vi "Get Control Offsets by Name.vi"(6 "offset":i32, 8 "error in (no error)":errorcluster, 9 "Controls":string[](array[string]), 10 "Indicators":string[](array[string]), 11 "bitfile xml in":string) -> (0 "error out":errorcluster, 1 "Control Offsets":T1[](array[typedef]), 2 "Indicator Offsets":T1[](array[typedef]), 4 "offset past EndTag":i32)   [LabVIEW 2010, in "FPGA Bitfile Utility.lvlib"]
uses:
  <userlib>/_FPGA Interface Advanced Tools/FPGA Bitfile Utility/FPGA Bitfile Utility.lvlib
  <userlib>/_FPGA Interface Advanced Tools/FPGA Bitfile Utility/TypeDefs/Control_Indicator Info.ctl
  <vilib>/rvi/DataTransferAndStorage/Container/Common/niFpgaDataTypeControl.ctl
  <userlib>/_FPGA Interface Advanced Tools/FPGA Bitfile Utility/Get Register Map.vi
  <userlib>/_FPGA Interface Advanced Tools/FPGA Bitfile Utility/Get Base Address.vi
  <vilib>/rvi/Utilities/XML/nirviXML_GetValue.vi
  <vilib>/rvi/Utilities/XML/nirviXML_GetValue_String.vi
  <vilib>/rvi/Bitfile/niFpgaReadBitfileXml_VIRegisterMap.vi
  <vilib>/rvi/Utilities/XML/nirviXML_GetValue_U32.vi
  <vilib>/Utility/VariantDataType/GetTypeInfo.vi
  <vilib>/Utility/VariantDataType/GetArrayInfo.vi
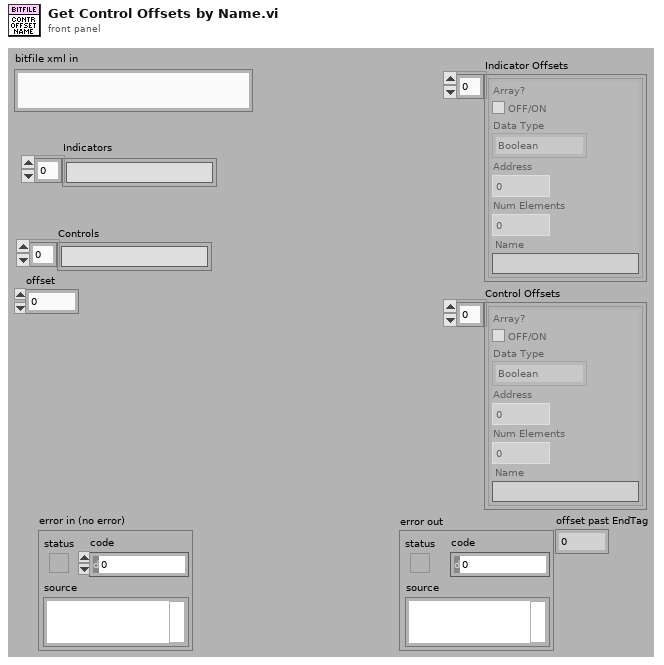
[diagram p1: front panel]
types:
  T1 = typedef "FPGA Bitfile Utility.lvlib/Control_Indicator Info.ctl" = cluster{"Array?":bool, "Data Type":T2, "Address":u32, "Num Elements":u32, "Name":string}
  T2 = typedef "niFpgaDataTypeControl.ctl" = enum32{"Boolean", "I8", "I16", "I32", "I64", "U8", "U16", "U32", "U64", "FXP", "CustomControl"}
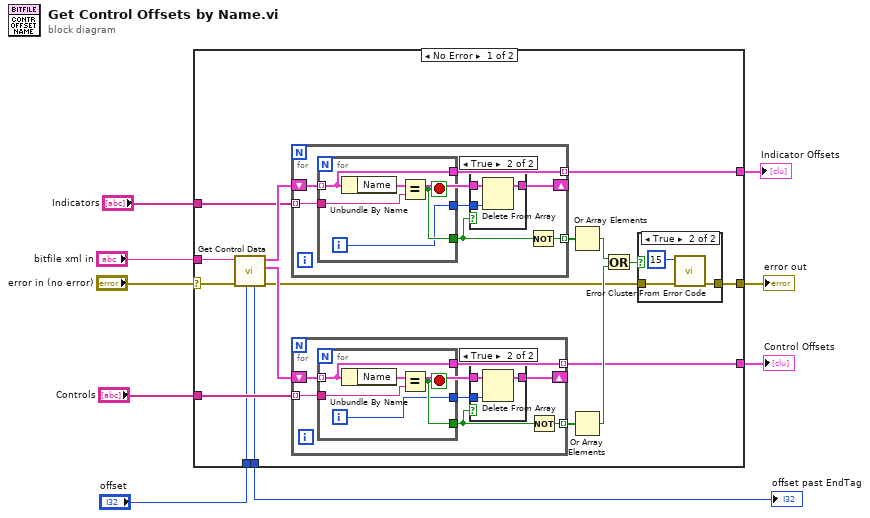
[diagram p0: block diagram]
diagram:
  n1 = case shown="No Error" "error in (no error)" {
    selector: "error in (no error)" -> [w26 w64]
    tunnel: "Controls" -> [w21 _]
    tunnel: [w11 _] -> w7
    tunnel: [w16 w64] -> w6
    tunnel: [w10 _] -> w4
    tunnel: "Indicators" -> [w15 _]
    tunnel: "bitfile xml in" -> [w14 _]
    tunnel: "offset" -> [w13 w63]
    tunnel: [w12 w63] -> w1
    frame No Error {
      n2 = call <userlib>:"Get Control Data.vi"("offset"=w13, "error in (no error)"=w26, "bitfile xml in"=w14) -> ("error out"=w17:errorcluster, "Controls"=w22:T1[], "Indicators"=w25:T1[], "offset past EndTag"=w12:i32)  [unwired: 5 in]
      n3 = for {
        tunnel: w15 -> [w53] mode=indexing
        tunnel: [w52] -> w11 mode=indexing
        tunnel: [w51] -> w24 mode=indexing
        shift-right: [w50] -> _
        shift-left: w25 -> [w48]
        n4 = for {
          tunnel: w48 -> [w60] mode=indexing
          tunnel: w53 -> [w61]
          tunnel: [w60] -> w52
          tunnel: [w59] -> w47
          tunnel: [w58] -> w49
          i -> [w58]
          stop <- w59 stop-if-true
          n5 = Unbundle By Name(w60) -> ("Name"=w62:string)
          n6 = Equal?(x=w62, y=w61) -> (x = y?=w59:bool)
        }
        n7 = case shown="True" w47 {
          tunnel: w48 -> [w54 w57]
          tunnel: [w54 w56] -> w50
          tunnel: w49 -> [_ w55]
          frame False {
          }
          frame True {
            n8 = Delete From Array(array=w57, index=w55) -> (array with subset deleted=w56:T1[])  [unwired: 1 in, 1 out]
          }
        }
        n9 = Not(x=w47) -> (.not. x?=w51:bool)
      }
      n10 = for {
        tunnel: w21 -> [w37] mode=indexing
        tunnel: [w36] -> w10 mode=indexing
        tunnel: [w35] -> w23 mode=indexing
        shift-right: [w33] -> _
        shift-left: w22 -> [w34]
        n11 = for {
          tunnel: w34 -> [w44] mode=indexing
          tunnel: w37 -> [w45]
          tunnel: [w44] -> w36
          tunnel: [w43] -> w31
          tunnel: [w42] -> w32
          i -> [w42]
          stop <- w43 stop-if-true
          n12 = Unbundle By Name(w44) -> ("Name"=w46:string)
          n13 = Equal?(x=w46, y=w45) -> (x = y?=w43:bool)
        }
        n14 = case shown="True" w31 {
          tunnel: w34 -> [w38 w41]
          tunnel: [w38 w40] -> w33
          tunnel: w32 -> [_ w39]
          frame False {
          }
          frame True {
            n15 = Delete From Array(array=w41, index=w39) -> (array with subset deleted=w40:T1[])  [unwired: 1 in, 1 out]
          }
        }
        n16 = Not(x=w31) -> (.not. x?=w35:bool)
      }
      n17 = Or Array Elements(Boolean array=w24) -> (logical OR=w20:bool)
      n18 = Or Array Elements(Boolean array=w23) -> (logical OR=w19:bool)
      n19 = Or(x=w20, y=w19) -> (x .or. y?=w18:bool)
      n20 = case shown="True" w18 {
        tunnel: w17 -> [w27 w29]
        tunnel: [w27 w28] -> w16
        frame False {
        }
        frame True {
          n21 = call <vilib>:"Error Cluster From Error Code.vi"("error in (no error)"=w29, "error code (0)"=15) -> ("error out"=w28:errorcluster)  [unwired: 7 in]
        }
      }
    }
    frame Error {
    }
  }
  "Control Offsets" <- w4
  "Indicator Offsets" <- w7
  "error out" <- w6
  "offset past EndTag" <- w1
